vi "Sequencer.vi"(8 "error in (no error)":errorcluster) -> (0 "Error State":errorcluster)   [LabVIEW 2017]
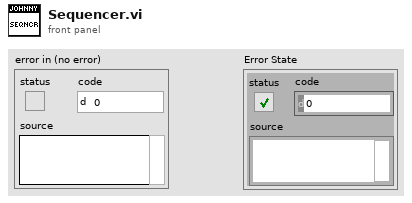
[diagram p1: front panel]
types:
  T1 = cluster{"Error State":errorcluster, "State_ndx":i32, "Timeout [s]":dbl}
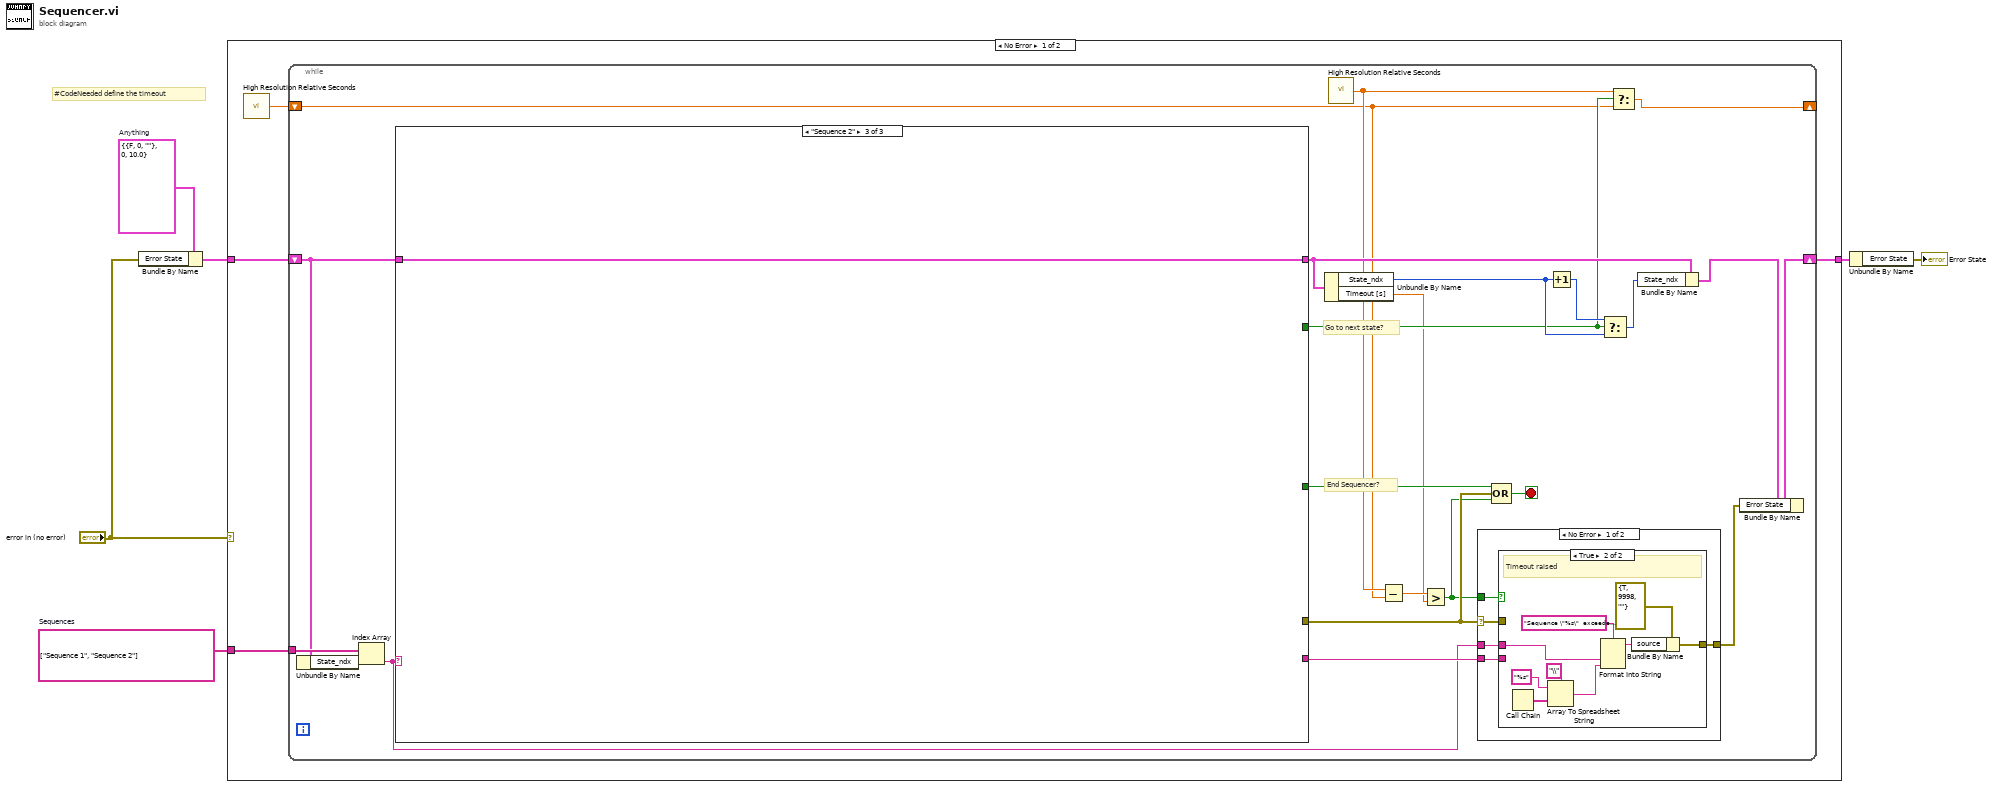
[diagram p0: block diagram]
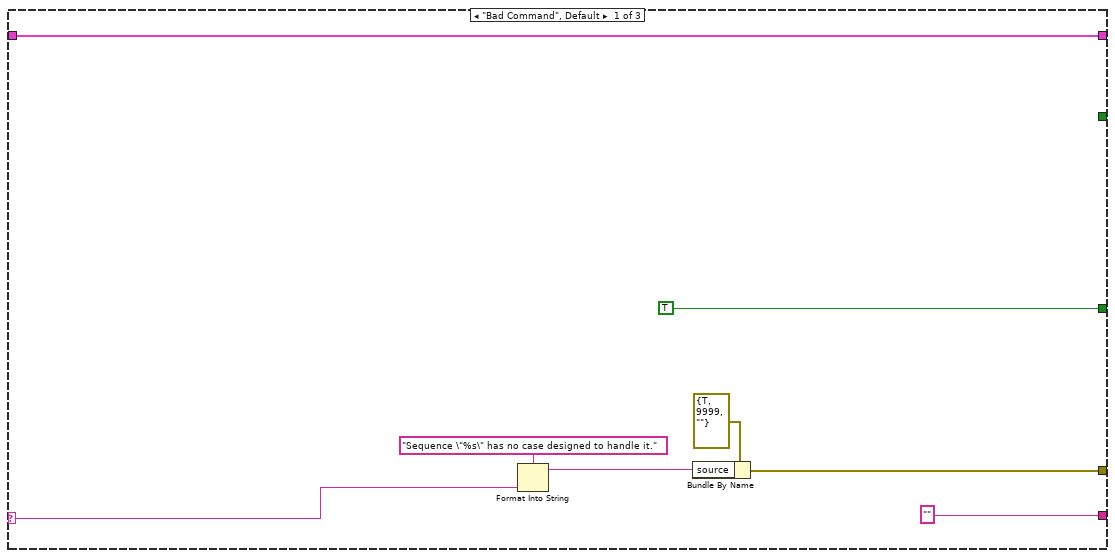
[diagram p2: hidden frame]
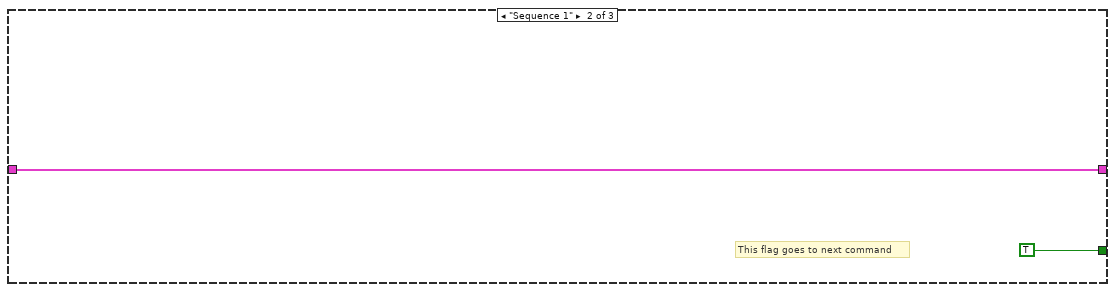
[diagram p3: hidden frame]
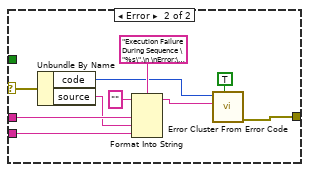
[diagram p5: hidden frame]
diagram:
  w2 = T1 {"Error State"={"status"=FALSE, "code"=0, "source"=""}, "State_ndx"=0, "Timeout [s]"=10.0}  # Anything
  w5 = string[] ["Sequence 1", "Sequence 2"]  # Sequences
  # "#CodeNeeded define the timeout"
  n1 = Bundle By Name(cluster=w2, "Error State"="error in (no error)") -> (w6:T1)
  n2 = case shown="No Error" "error in (no error)" {
    tunnel: w5 -> [w10 _]
    tunnel: w6 -> [w9 w69]
    tunnel: [w8 w69] -> w3
    frame No Error {
      n3 = call <vilib>:"High Resolution Relative Seconds.vi"() -> ("relative seconds"=w7:dbl)
      n4 = while {
        tunnel: w10 -> [w31]
        shift-right: [w32] -> w8
        shift-left: w9 -> [w27]
        shift-right: [w15] -> _
        shift-left: w7 -> [w16]
        stop <- w19 stop-if-true
        # "End Sequencer?"
        # "Go to next state?"
        n5 = Unbundle By Name(w27) -> ("State_ndx"=w26:i32)
        n6 = Index Array(array=w31, index=w26) -> (element=w28:string)
        n7 = case shown="\"Sequence 2\"" w28 {
          selector: w28 -> [w35 _ _]
          tunnel: w27 -> [w40 w42 w43]
          tunnel: [w40 w42 w43] -> w24
          tunnel: [w37 _ _] -> w12
          tunnel: ["" ("Accessors:Name") _ _] -> w30
          tunnel: [_ TRUE ("s") _] -> w18
          tunnel: [TRUE _ _] -> w20
          frame "Bad Command", Default {
            n8 = Format Into String(format string="Sequence \"%s\" has no case designed to handle it.", w35) -> (resulting string=w34:string)  [unwired: 2 in, 1 out]
            n9 = Bundle By Name(cluster=errorcluster {"status"=TRUE, "code"=9999, "source"=""} ("error out"), "source"=w34) -> (w37:errorcluster)
          }
          frame "Sequence 1" {
            # "This flag goes to next command"
          }
          frame "Sequence 2" {
          }
        }
        n10 = Unbundle By Name(w24) -> ("State_ndx"=w21:i32, "Timeout [s]"=w13:dbl)
        n11 = call <vilib>:"High Resolution Relative Seconds.vi"() -> ("relative seconds"=w17:dbl)
        n12 = Subtract(x=w17, y=w16) -> (x-y=w14:dbl)
        n13 = Greater?(x=w14, y=w13) -> (0:w11:bool)
        n14 = case shown="No Error" w12 {
          selector: w12 -> [w46 w62]
          tunnel: [w47 w67] -> w29
          tunnel: w28 -> [w45 w65]
          tunnel: w30 -> [w44 w60]
          tunnel: w11 -> [w48 _]
          frame No Error {
            n15 = case shown="True" w48 {
              tunnel: w45 -> [_ w57]
              tunnel: [w49 w54] -> w47
              tunnel: w46 -> [w49 _]
              tunnel: w44 -> [_ _]
              frame False {
              }
              frame True {
                # "Timeout raised"
                n16 = Call Chain() -> (call chain=w53:string[])
                n17 = Array To Spreadsheet String(delimiter (Tab)="\\", array=w53, 3:"%s") -> (spreadsheet string=w50:string)
                n18 = Format Into String(format string="Sequence \"%s\"  exceeded the timeout.\n\n%s" ("source"), w57, w50) -> (resulting string=w55:string)  [unwired: 2 in, 1 out]
                n19 = Bundle By Name(cluster=errorcluster {"status"=TRUE, "code"=9998, "source"=""} ("error out"), "source"=w55) -> (w54:errorcluster)
              }
            }
          }
          frame Error {
            n20 = Unbundle By Name(w62) -> ("code"=w59:i32, "source"=w61:string)
            n21 = Format Into String(format string="Execution Failure During Sequence \"%s\".\n \nError:\n%s\n\n%s" ("error message (\"\")"), initial string="", w65, w61, w60) -> (resulting string=w66:string)  [unwired: 1 in, 1 out]
            n22 = call <vilib>:"Error Cluster From Error Code.vi"("show call chain? (False)"=TRUE, "error message (\"\")"=w66, "error code (0)"=w59) -> ("error out"=w67:errorcluster)  [unwired: 6 in]
          }
        }
        n23 = Compound Arithmetic op=OR(w20, w12, w11) -> (w19:bool)
        n24 = Increment(x=w21) -> (x+1=w23:i32)
        n25 = Select(t=w23, s=w18, f=w21) -> (s? t:f=w22:i32)
        n26 = Select(t=w17, s=w18, f=w16) -> (s? t:f=w15:dbl)
        n27 = Bundle By Name(cluster=w24, "State_ndx"=w22) -> (w25:T1)
        n28 = Bundle By Name(cluster=w25, "Error State"=w29) -> (w32:T1)
      }
    }
    frame Error {
    }
  }
  n29 = Unbundle By Name(w3) -> ("Error State"=→"Error State":errorcluster)
